vi "多参数 interface.vi"(8 "error in (no error)":errorcluster caption="错误输入（无错误）") -> ()   [LabVIEW 2016, in "斯坦道多参数.lvlib"]
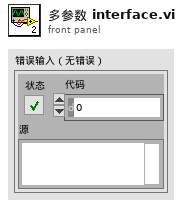
[diagram p1: front panel]
types:
  T1 = typedef "多参数交互.ctl" = cluster{"pH":bool, "DO":bool, "Turb":bool, "Cond":bool, "Temp":bool, "叶绿素a启用":bool, "蓝绿藻":bool, "藻密度":bool, "orp":bool}
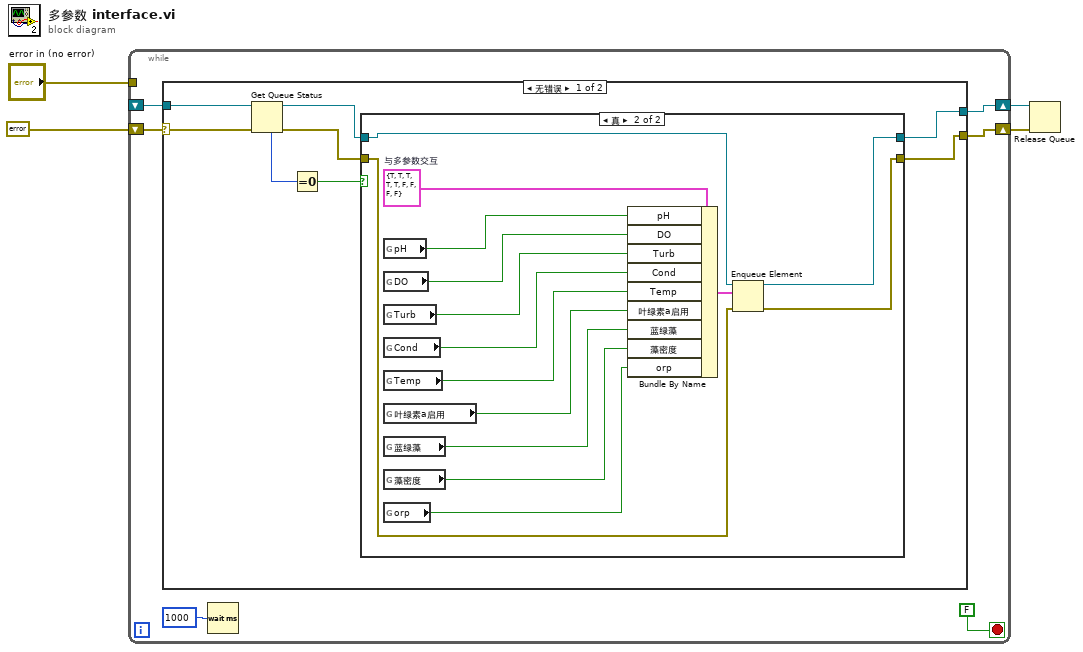
[diagram p0: block diagram]
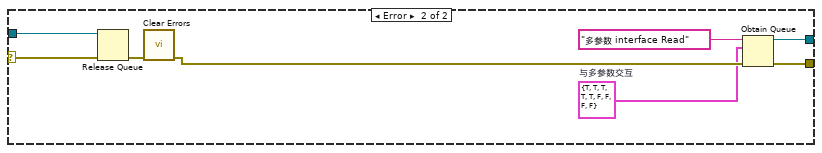
[diagram p3: hidden frame]
diagram:
  n1 = while {
    shift-right: [w10] -> w2
    shift-left: errorcluster {"status"=TRUE, "code"=0, "source"=""} ("error out") -> [w9]
    shift-right: [w8] -> w3
    shift-left: _ -> [w7]
    tunnel: "error in (no error)" -> [_]
    stop <- FALSE stop-if-true
    n2 = case shown="无错误" w9 {
      selector: w9 -> [w14 w40]
      tunnel: [w16 w42] -> w10
      tunnel: [w17 w41] -> w8
      tunnel: w7 -> [w18 w39]
      frame No Error {
        n3 = Get Queue Status(queue=w18, error in (no error)=w14) -> (queue out=w15:refnum<queue>, error out=w13:errorcluster, # elements in queue=w12:i32)  [unwired: 1 in, 5 out]
        n4 = Equal To 0?(x=w12) -> (x = 0?=w11:bool)
        n5 = case shown="真" w11 {
          tunnel: [w20 w35] -> w17
          tunnel: [w19 w34] -> w16
          tunnel: w15 -> [w20 w22]
          tunnel: w13 -> [w19 w21]
          frame False {
          }
          frame True {
            w33 = T1 {"pH"=TRUE, "DO"=TRUE, "Turb"=TRUE, "Cond"=TRUE, "Temp"=TRUE, "叶绿素a启用"=FALSE, "蓝绿藻"=FALSE, "藻密度"=FALSE, "orp"=FALSE}  # 与多参数交互
            n6 = global read "断电保存变量.vi" "pH"() -> (w32:bool)
            n7 = global read "断电保存变量.vi" "DO"() -> (w31:bool)
            n8 = global read "断电保存变量.vi" "Turb"() -> (w30:bool)
            n9 = global read "断电保存变量.vi" "Cond"() -> (w29:bool)
            n10 = global read "断电保存变量.vi" "Temp"() -> (w28:bool)
            n11 = global read "断电保存变量.vi" "叶绿素a启用"() -> (w27:bool)
            n12 = global read "断电保存变量.vi" "蓝绿藻"() -> (w26:bool)
            n13 = global read "断电保存变量.vi" "藻密度"() -> (w25:bool)
            n14 = global read "断电保存变量.vi" "orp"() -> (w24:bool)
            n15 = Bundle By Name(cluster=w33, "pH"=w32, "DO"=w31, "Turb"=w30, "Cond"=w29, "Temp"=w28, "叶绿素a启用"=w27, "蓝绿藻"=w26, "藻密度"=w25, "orp"=w24) -> (w23:T1)
            n16 = Enqueue Element(queue=w22, element=w23, error in (no error)=w21) -> (queue out=w35:refnum<queue>, error out=w34:errorcluster)  [unwired: 1 in, 1 out]
          }
        }
      }
      frame Error {
        w36 = T1 {"pH"=TRUE, "DO"=TRUE, "Turb"=TRUE, "Cond"=TRUE, "Temp"=TRUE, "叶绿素a启用"=FALSE, "蓝绿藻"=FALSE, "藻密度"=FALSE, "orp"=FALSE}  # 与多参数交互
        n17 = Release Queue(queue=w39, error in (no error)=w40) -> (error out=w38:errorcluster)  [unwired: 1 in, 2 out]
        n18 = call <vilib>:"Clear Errors.vi"("error in (no error)"=w38) -> ("error out"=w37:errorcluster)  [unwired: 5 in, 1 out]
        n19 = Obtain Queue(name (unnamed)="多参数 interface Read" ("写入方名称"), element data type=w36, error in (no error)=w37) -> (queue out=w41:refnum<queue>, error out=w42:errorcluster)  [unwired: 2 in, 1 out]
      }
    }
    n20 = Wait (ms)(milliseconds to wait=u32 1000 ("等待时间（毫秒）")) -> ()  [unwired: 1 out]
  }
  n21 = Release Queue(queue=w3, error in (no error)=w2) -> ()  [unwired: 1 in, 3 out]
